vi "Insert_2Event_Log(Classify).vi"(6 "account":string="B", 7 "classify":i16=1, 8 "data":string="790", 9 "message":string="B", 10 "output cluster":cluster{"barcode A":string, "barcode B":string}, 11 "DBlink":string="Driver={ODBC Driver 17 for SQL Server};Server=localhost\\SQLEXPRESS;Database=ZDX201;UID=labview;PWD=Dsa@54137926") -> ()   [LabVIEW 2019]
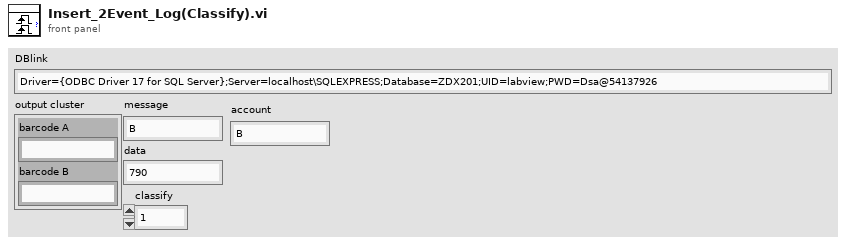
[diagram p1: front panel]
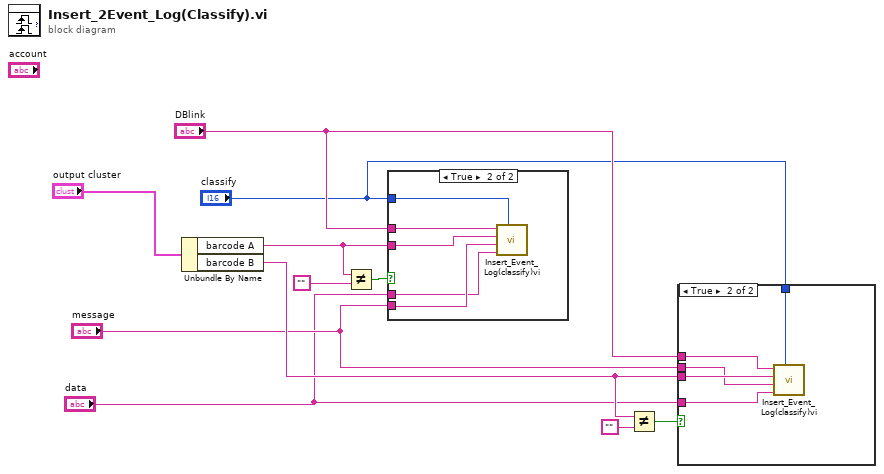
[diagram p0: block diagram]
diagram:
  n1 = Unbundle By Name("output cluster") -> ("barcode A"=w7:string, "barcode B"=w6:string)
  n2 = Not Equal?(x=w7, y="") -> (x != y?=w8:bool)
  n3 = case shown="True" w8 {
    tunnel: "DBlink" -> [_ w16]
    tunnel: w7 -> [_ w15]
    tunnel: "message" -> [_ w14]
    tunnel: "data" -> [_ w13]
    tunnel: "classify" -> [_ w12]
    frame False {
    }
    frame True {
      n4 = call "Insert_Event_Log(classify)vi.vi"("classify"=w12, "data"=w13, "message"=w14, "id"=w15, "DBlink"=w16) -> ()  [unwired: 6 in, 1 out]
    }
  }
  n5 = Not Equal?(x=w6, y="") -> (x != y?=w4:bool)
  n6 = case shown="True" w4 {
    tunnel: w6 -> [_ w20]
    tunnel: "DBlink" -> [_ w21]
    tunnel: "message" -> [_ w19]
    tunnel: "data" -> [_ w18]
    tunnel: "classify" -> [_ w17]
    frame False {
    }
    frame True {
      n7 = call "Insert_Event_Log(classify)vi.vi"("classify"=w17, "data"=w18, "message"=w19, "id"=w20, "DBlink"=w21) -> ()  [unwired: 6 in, 1 out]
    }
  }
